vi "read_string_lines.vi"() -> ()   [LabVIEW 2021]
panel:
  out "string array":string[](array[string])
  out "path":path
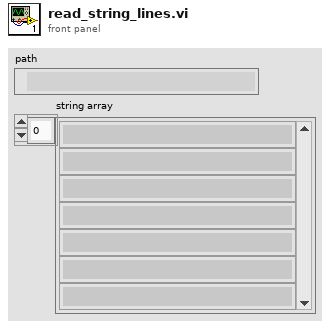
[diagram p1: front panel]
types:
  T1 = enum16{"open", "replace", "create", "open or create", "replace or create", "replace or create with confirmation"}
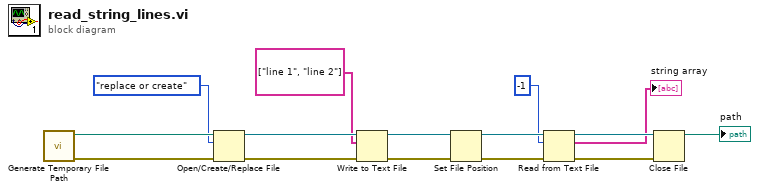
[diagram p0: block diagram]
diagram:
  n1 = call <vilib>:"Generate Temporary File Path.vi"() -> ("error out"=w5:errorcluster, "Unique Temporary File Path"=w6:path)  [unwired: 10 in]
  n2 = Open/Create/Replace File(file path (use dialog)=w6, error in=w5, operation (0:open)=T1."replace or create") -> (refnum out=w7:refnum<file>, error out=w9:errorcluster)  [unwired: 3 in, 1 out]
  n3 = Write to Text File(file (use dialog)=w7, text=string[] ["line 1", "line 2"], error in=w9) -> (refnum out=w8:refnum<file>, error out=w10:errorcluster)  [unwired: 1 in, 1 out]
  n4 = Set File Position(refnum=w8, error in=w10) -> (refnum out=w11:refnum<file>, error out=w12:errorcluster)  [unwired: 2 in]
  n5 = Read from Text File(file (use dialog)=w11, count=-1, error in=w12) -> (refnum out=w14:refnum<file>, text=→"string array":string[], error out=w13:errorcluster)  [unwired: 1 in, 1 out]
  n6 = Close File(refnum=w14, error in=w13) -> (path=→"path":path)  [unwired: 1 out]
